vi "_Set UserEvent.vi"(8 "error in (no error)":errorcluster, 10 "UserEvent":refnum<user-event>, 11 "Event in":refnum<class "Event.lvclass">) -> (0 "error out":errorcluster, 3 "Event out":refnum<class "Event.lvclass">)   [LabVIEW 2009, in "EventManagerLibrary.lvlib" / "Event.lvclass"]
uses:
  Event.lvclass
  EventDataObject/EventData.lvclass
  Event.lvclass/Event.ctl
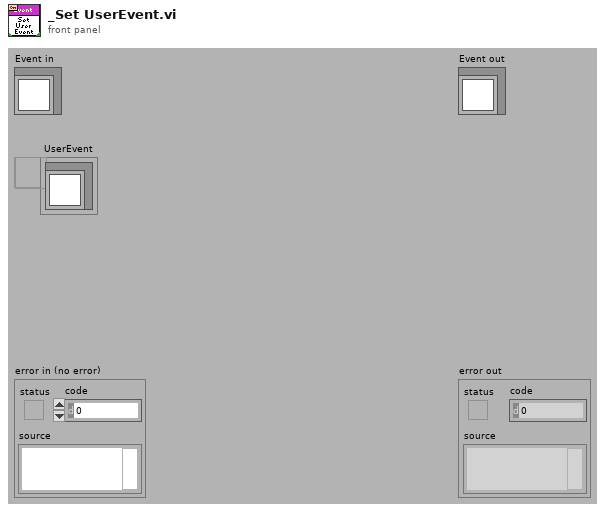
[diagram p1: front panel]
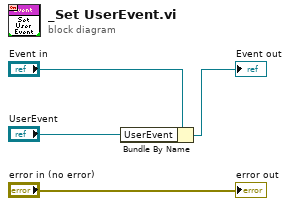
[diagram p0: block diagram]
diagram:
  n1 = Bundle By Name(cluster="Event in", "UserEvent"="UserEvent") -> (→"Event out":refnum<class "Event.lvclass">)
  "error out" <- "error in (no error)"
